vi "State Exit.vi"(8 "error in (no error)":errorcluster, 11 "View Model":T1) -> (0 "error out":errorcluster, 3 "View Model":T1)   [LabVIEW 2017]
doc: "Handle state transitions"
uses:
  View Model/Controls/View Model.ctl
  Error Handler/Controls/Error Model.ctl
  Error Handler/Controls/Error EventData.ctl
  Error Handler/Controls/Error Type.ctl
  Controls/Elevator Model.ctl
  Controls/Elevator Overhead.ctl
  Controls/Elevator States.ctl
  Controls/Elevator Location.ctl
  Controls/Elevator Command Event.ctl
  Controls/Elevator Commands.ctl
  Configuration/Controls/Configuration Model.ctl
  Configuration/Controls/Configuration Data.ctl
  View Model/Controls/Shared Model.ctl
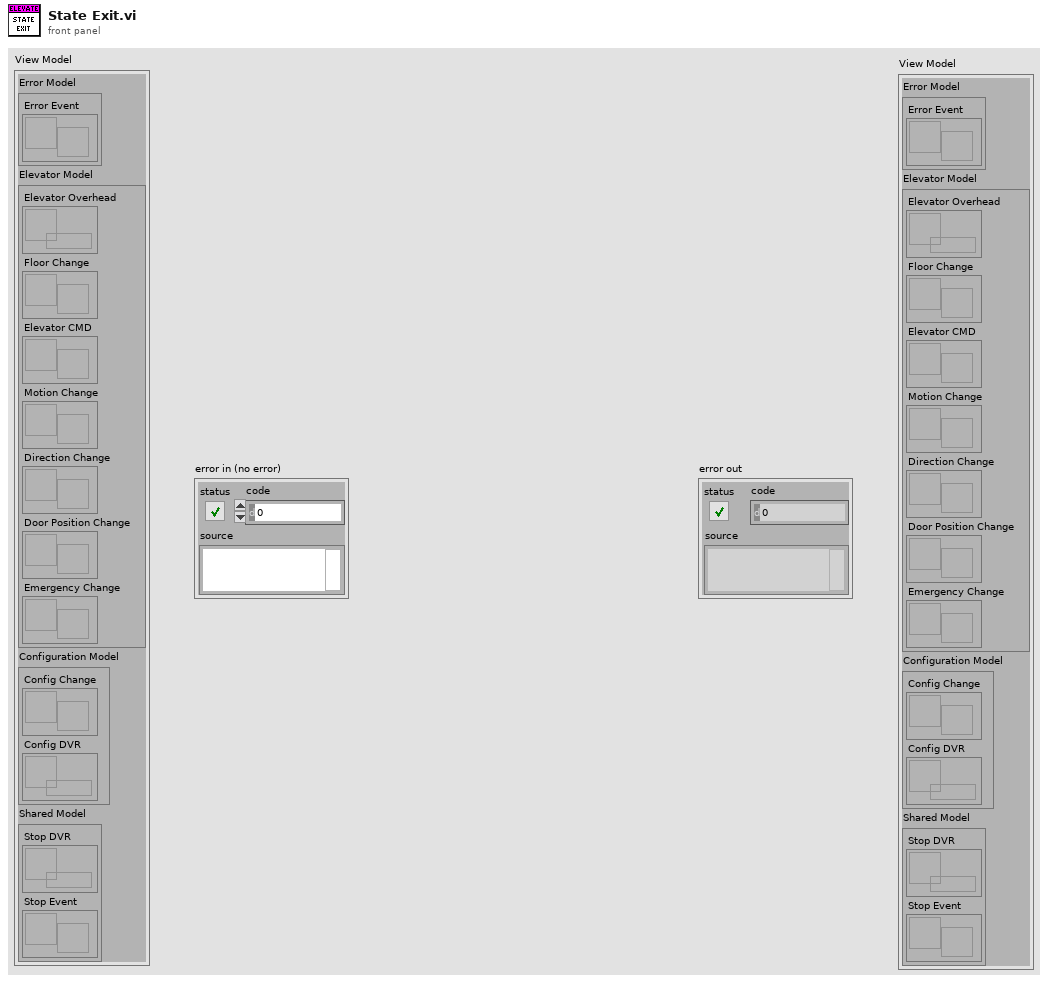
[diagram p1: front panel]
types:
  T1 = typedef "View Model.ctl" = cluster{"Error Model":T2, "Elevator Model":T3, "Configuration Model":T4, "Shared Model":T5}
  T2 = typedef "Error Model.ctl" = cluster{"Error Event":refnum<user-event>}
  T3 = typedef "Elevator Model.ctl" = cluster{"Elevator Overhead":refnum<data-value>, "Floor Change":refnum<user-event>, "Elevator CMD":refnum<user-event>, "Motion Change":refnum<user-event>, "Direction Change":refnum<user-event>, "Door Position Change":refnum<user-event>, "Emergency Change":refnum<user-event>}
  T4 = typedef "Configuration Model.ctl" = cluster{"Config Change":refnum<user-event>, "Config DVR":refnum<data-value>}
  T5 = typedef "Shared Model.ctl" = cluster{"Stop DVR":refnum<data-value>, "Stop Event":refnum<user-event>}
  T6 = typedef "Elevator States.ctl" = enum16{"Idle", "Init", "Open Doors", "Close Doors", "Start Move", "Move", "Finish Move", "Analysis", "Emergency"}
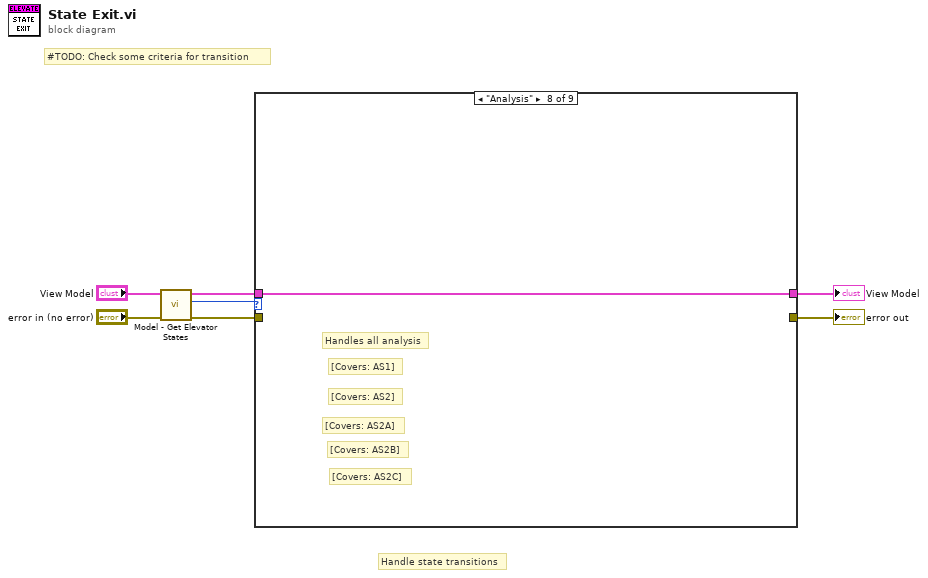
[diagram p0: block diagram]
diagram:
  # "Handle state transitions"
  # "#TODO: Check some criteria for transition"
  n1 = call "Model - Get Elevator States.vi"("error in (no error)"="error in (no error)", "View Model"="View Model") -> ("error out"=w3:errorcluster, "Elevator State"=w4:T6, "View Model"=w5:T1)  [unwired: 6 in, 1 out]
  n2 = case shown="\"Analysis\"" w4 {
    tunnel: w5 -> [w9 w10 w11 w12 w13 w14 w15 w16 w17]
    tunnel: w3 -> [w8 _ _ _ _ _ _ _ _]
    tunnel: [w9 w10 w11 w12 w13 w14 w15 w16 w17] -> w2
    tunnel: [w8 _ _ _ _ _ _ _ _] -> w1
    frame "Idle", Default {
    }
    frame "Init" {
      # "[Covers: NR1A]"
      # "If inactivity timer <=0, transition to start move with 1st floor as destination"
    }
    frame "Open Doors" {
      # "[Covers: OC3B]"
      # "If open door timer <=0, go to close state"
    }
    frame "Close Doors" {
      # "[Covers: OC7]"
      # "Transition to initial state"
    }
    frame "Start Move" {
    }
    frame "Move" {
      # "[Covers: CT1B]"
      # "[Covers: SS4B]"
      # "If time has elapsed, stop elevator. Update floor position"
    }
    frame "Finish Move" {
      # "[Covers: RF3]"
      # "Transition to door open/close"
    }
    frame "Analysis" {
      # "[Covers: AS2C]"
      # "[Covers: AS2B]"
      # "[Covers: AS2A]"
      # "[Covers: AS2]"
      # "[Covers: AS1]"
      # "Handles all analysis"
    }
    frame "Emergency" {
    }
  }
  "View Model" <- w2
  "error out" <- w1
